vi "Scale Graphs.vi"(8 "error in (no error)":errorcluster, 11 "Detail Graph in":refnum<class "Detail Graph.lvclass">) -> (0 "error out":errorcluster, 3 "Detail Graph out":refnum<class "Detail Graph.lvclass">)   [LabVIEW 2023, in "Detail Graph.lvclass"]
uses:
  Detail Graph.lvclass
  Detail Graph.lvclass/Detail Graph.ctl
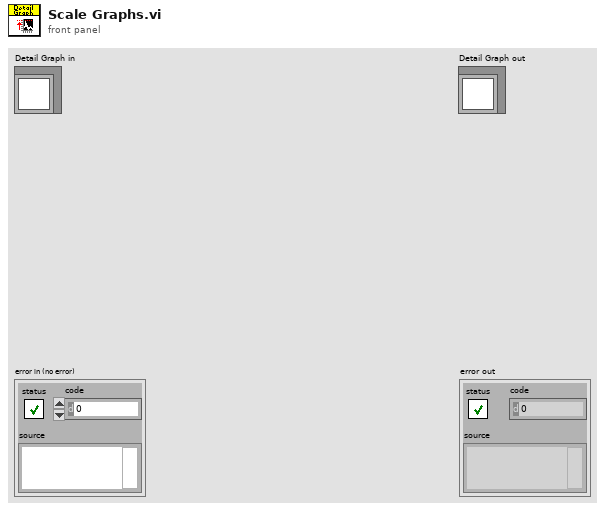
[diagram p1: front panel]
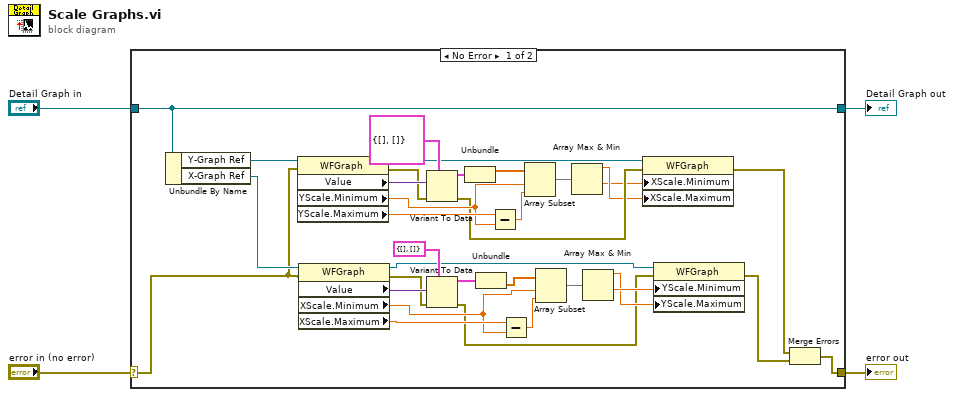
[diagram p0: block diagram]
diagram:
  n1 = case shown="No Error" "error in (no error)" {
    selector: "error in (no error)" -> [w20 w39]
    tunnel: [w22 w39] -> w3
    tunnel: [w37 w38] -> w1
    tunnel: "Detail Graph in" -> [w37 w38]
    frame No Error {
      n2 = Unbundle By Name(w37) -> ("Y-Graph Ref"=w36:refnum<vi>, "X-Graph Ref"=w21:refnum<vi>)
      n3 = property class="WFGraph"(reference=w36, error in=w20) -> (reference out=w27:refnum<vi>, error out=w28:errorcluster, "Value"=w35:variant, "YScale.Minimum"=w30:dbl, "YScale.Maximum"=w31:dbl)
      n4 = property class="WFGraph"(reference=w21, error in=w20) -> (reference out=w13:refnum<vi>, error out=w9:errorcluster, "Value"=w18:variant, "XScale.Minimum"=w11:dbl, "XScale.Maximum"=w12:dbl)
      n5 = Variant To Data(error in=w28, type=cluster{dbl[], dbl[]} {[], []} ("cluster"), Variant=w35) -> (data=w33:cluster{dbl[], dbl[]}, error out=w26:errorcluster)
      n6 = Variant To Data(error in=w9, type=cluster{dbl[], dbl[]} {[], []} ("cluster"), Variant=w18) -> (data=w6:cluster{dbl[], dbl[]}, error out=w10:errorcluster)
      n7 = Unbundle(w33) -> (w32:dbl[])  [unwired: 1 out]
      n8 = Unbundle(w6) -> (w5:dbl[])  [unwired: 1 out]
      n9 = Subtract(x=w31, y=w30) -> (x-y=w29:dbl)
      n10 = Subtract(x=w12, y=w11) -> (x-y=w14:dbl)
      n11 = Array Subset(array=w32, index=w30, length=w29) -> (w25:dbl[])
      n12 = Array Subset(array=w5, index=w11, length=w14) -> (w15:dbl[])
      n13 = Array Max & Min(array=w25) -> (max value=w24:dbl, min value=w23:dbl)  [unwired: 2 out]
      n14 = Array Max & Min(array=w15) -> (max value=w16:dbl, min value=w17:dbl)  [unwired: 2 out]
      n15 = property class="WFGraph"(reference=w27, error in=w26, "XScale.Minimum"=w23, "XScale.Maximum"=w24) -> (error out=w7:errorcluster)  [unwired: 1 out]
      n16 = property class="WFGraph"(reference=w13, error in=w10, "YScale.Minimum"=w17, "YScale.Maximum"=w16) -> (error out=w8:errorcluster)  [unwired: 1 out]
      n17 = Merge Errors(w7, w8) -> (w22:errorcluster)
    }
    frame Error {
    }
  }
  "error out" <- w3
  "Detail Graph out" <- w1
